vi "Get All Environment Variables [Map].vi"(7 "Target (Process)":T1 items=["Process", "User", "Machine"], 8 "Error In":errorcluster) -> (0 "Error Out":errorcluster, 3 "Variables":map{string, string}(c390))   [LabVIEW 2023, in "SLL Environment Variable.lvlib"]
doc: "Retrieve all environment variables and their values from the target environment in a map."
uses:
  SLL Environment Variable.lvlib
  _Typedef/Target Environment Enum.ctl
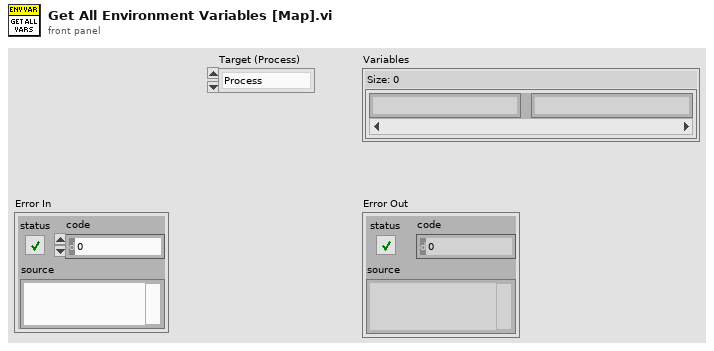
[diagram p1: front panel]
types:
  T1 = typedef "SLL Environment Variable.lvlib/Target Environment Enum.ctl" = i32
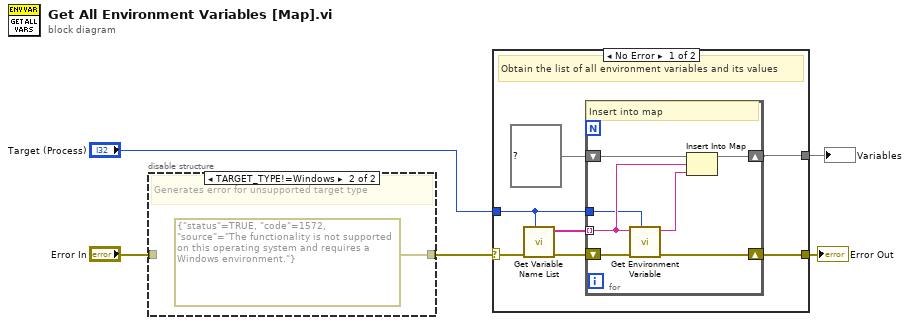
[diagram p0: block diagram]
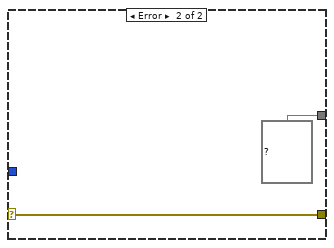
[diagram p3: hidden frame]
diagram:
  n1 = disable-structure shown="TARGET_TYPE!=Windows" {
    disable-tunnel: "Error In" -> [w6 _]
    disable-tunnel: [w6 errorcluster {"status"=TRUE, "code"=1572, "source"="The functionality is not supported on this operating system and requires a Windows environment."} ("Error In")] -> w2
    frame condition #0 (active) {
    }
    frame condition #1 {
      # "Generates error for unsupported target type"
    }
  }
  n2 = case shown="No Error" w2 {
    selector: w2 -> [w10 w23]
    tunnel: [w14 w23] -> w5
    tunnel: [w12 map{string, string} {} ("map in")] -> w4
    tunnel: "Target (Process)" -> [w8 _]
    frame No Error {
      # "Obtain the list of all environment variables and its values"
      n3 = call "Get Variable Name List.vi"("Target (Process)"=w8, "Error In"=w10) -> ("Error Out"=w11:errorcluster, "Names[]"=w9:string[])  [unwired: 8 in]
      n4 = for {
        shift-right: [w20] -> w14
        shift-left: w11 -> [w21]
        tunnel: w9 -> [w17] mode=indexing
        shift-right: [w18] -> w12
        shift-left: map{string, string} {} ("map in") -> [w19]
        tunnel: w8 -> [w15]
        # "Insert into map"
        n5 = call "Get Environment Variable.vi"("Target (Process)"=w15, "Error In"=w21, "Name"=w17) -> ("Error Out"=w20:errorcluster, "Value"=w16:string)  [unwired: 7 in]
        n6 = Insert Into Map(map in=w19, key=w17, value=w16) -> (map out=w18:map{string, string})  [unwired: 2 out]
      }
    }
    frame Error {
    }
  }
  "Error Out" <- w5
  "Variables" <- w4
